vi "Force Window.vi"   [LabVIEW 2014, in "NI_AALPro.lvlib"]
doc: "Applies a force window to the input signal <B>X</B>. Wire data to the <B>X</B> input to determine the polymorphic instance to use or manually select the instance."
uses:
  NI_AALPro.lvlib
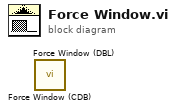
[diagram p0: block diagram]
diagram:
  n1 = call "Force Window (CDB).vi"() -> ()  [unwired: 2 in, 2 out]
  n2 = call "Force Window (DBL).vi"() -> ()  [unwired: 2 in, 2 out]
